vi "Time Profile Logger.vi"(6 "Flush and Close? (F)":bool, 7 "Initialize Settings":T1={"File Name"="SLL Time Profile Logger.txt", "Log Directory Path"=path "", "Initialize? (F)"=FALSE}, 8 "Error In":errorcluster, 9 "Tag Array":string[](array[string]), 10 "Tag 2":string, 11 "Tag 1":string) -> (0 "Error Out":errorcluster, 3 "Log Path":path)   [LabVIEW 2014, in "SLL Debug.lvlib"]
doc: "Simple Time Profile Logger with multiple tag inputs. \n\n<b>Important!</b> -The final call to this VI needs to have the \"Flush and Close?\" boolean set to log to file.\n\nDuring logging, the items are just put into a queue. Only during close operation, the data is parsed and logged to file. Supports logging into *.bin, *.csv & *.txt based on the file extension provided to the file name."
uses:
  SLL Debug.lvlib
  <vilib>/Utility/file.llb/Write To Spreadsheet File (string).vi
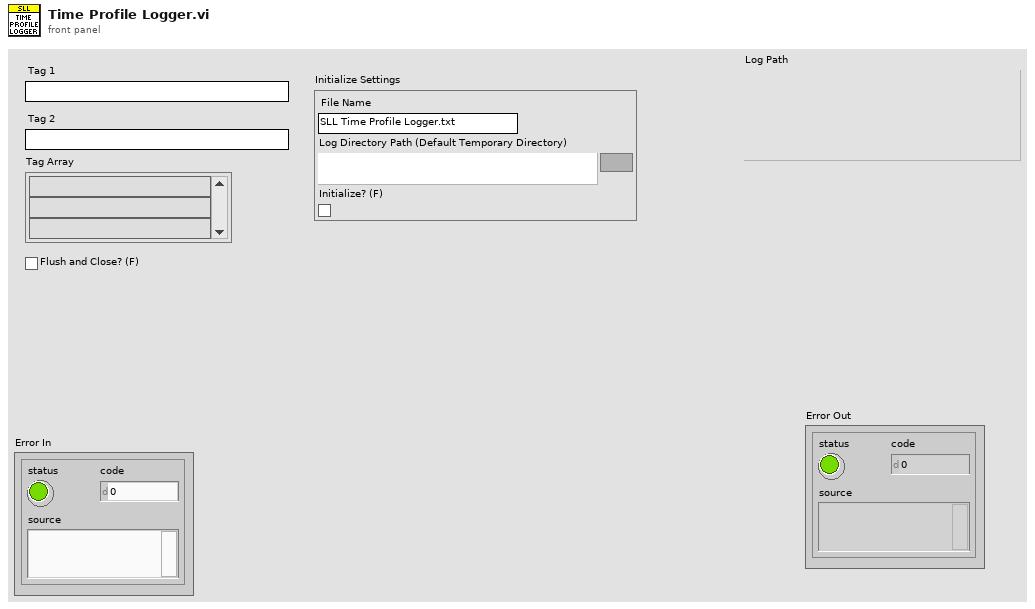
[diagram p1: front panel]
types:
  T1 = cluster{"File Name":string, "Log Directory Path":path, "Initialize? (F)":bool}
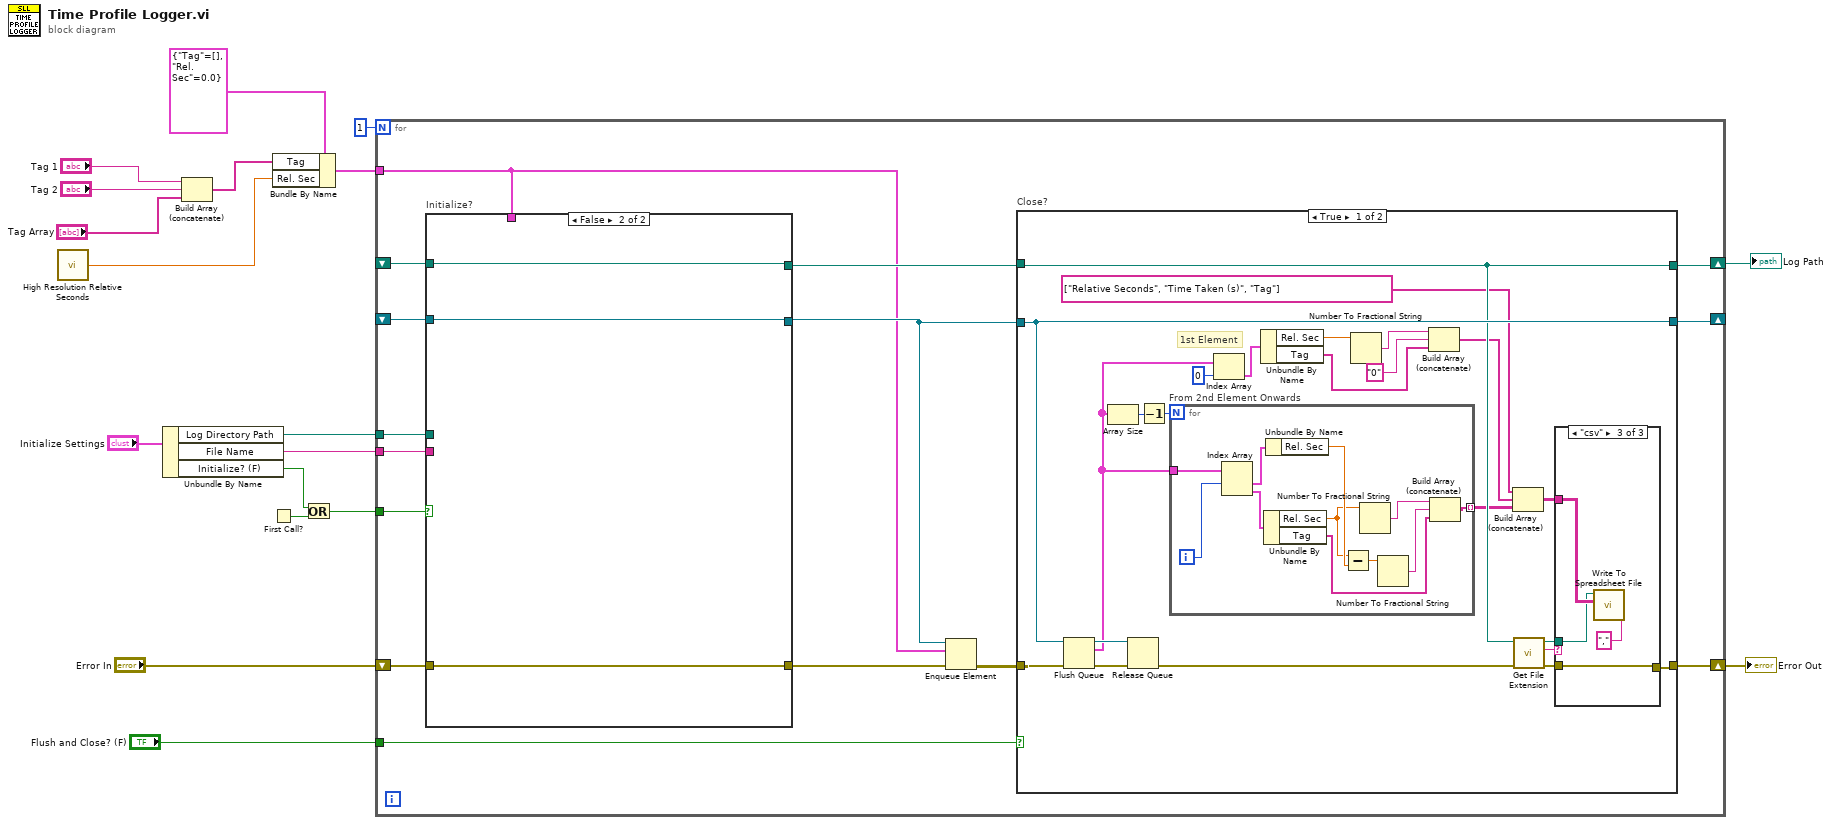
[diagram p0: block diagram]
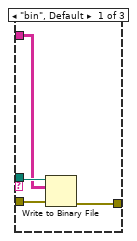
[diagram p2: hidden frame]
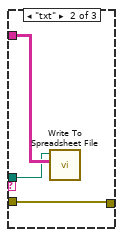
[diagram p3: hidden frame]
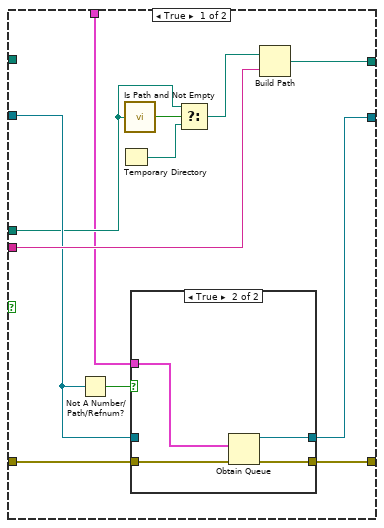
[diagram p5: hidden frame]
diagram:
  n1 = call <vilib>:"High Resolution Relative Seconds.vi"() -> ("relative seconds"=w2:dbl)
  n2 = Unbundle By Name("Initialize Settings") -> ("Log Directory Path"=w11:path, "File Name"=w10:string, "Initialize? (F)"=w6:bool)
  n3 = Build Array (concatenate)("Tag 1", "Tag 2", "Tag Array") -> (w4:string[])
  n4 = First Call?() -> (First Call?: T/F=w1:bool)
  n5 = Bundle By Name(cluster=cluster{"Tag":string[], "Rel. Sec":dbl} {"Tag"=[], "Rel. Sec"=0.0}, "Tag"=w4, "Rel. Sec"=w2) -> (w3:cluster{"Tag":string[], "Rel. Sec":dbl})
  n6 = Or(x=w6, y=w1) -> (x .or. y?=w9:bool)
  n7 = for {
    N: 1 -> [_]
    tunnel: w3 -> [w19]
    shift-right: [w20] -> w17
    shift-left: "Error In" -> [w33]
    shift-right: [w22] -> _
    shift-left: _ -> [w32]
    tunnel: w10 -> [w31]
    shift-right: [w21] -> w16
    shift-left: _ -> [w30]
    tunnel: w11 -> [w29]
    tunnel: w9 -> [w28]
    tunnel: "Flush and Close? (F)" -> [w27]
    n8 = case "Initialize?" shown="False" w28 {
      tunnel: w33 -> [w93 w102]
      tunnel: [w92 w102] -> w26
      tunnel: [w91 w101] -> w23
      tunnel: w32 -> [w87 w101]
      tunnel: w31 -> [w90 _]
      tunnel: [w89 w100] -> w24
      tunnel: w30 -> [_ w100]
      tunnel: w29 -> [w85 _]
      tunnel: w19 -> [w82 _]
      frame True {
        n9 = Not A Number/Path/Refnum?(number/path/refnum=w87) -> (NaN/Path/Refnum?=w88:bool)
        n10 = Temporary Directory() -> (w84:path)
        n11 = call <vilib>:"Is Path and Not Empty.vi"("path"=w85) -> ("Is Path and Not Empty?"=w86:bool)  [unwired: 4 in]
        n12 = case shown="True" w88 {
          tunnel: w93 -> [w94 w99]
          tunnel: [w94 w98] -> w92
          tunnel: [w95 w97] -> w91
          tunnel: w87 -> [w95 _]
          tunnel: w82 -> [_ w96]
          frame False {
          }
          frame True {
            n13 = Obtain Queue(element data type=w96, error in (no error)=w99) -> (queue out=w97:refnum<queue>, error out=w98:errorcluster)  [unwired: 3 in, 1 out]
          }
        }
        n14 = Select(t=w85, s=w86, f=w84) -> (s? t:f=w83:path)
        n15 = Build Path(base path=w83, name or relative path=w90) -> (appended path=w89:path)
      }
      frame False {
      }
    }
    n16 = Enqueue Element(queue=w23, element=w19, error in (no error)=w26) -> (error out=w25:errorcluster)  [unwired: 1 in, 2 out]
    n17 = case "Close?" shown="True" w27 {
      tunnel: w25 -> [w56 w81]
      tunnel: [w47 w81] -> w20
      tunnel: [w54 w80] -> w22
      tunnel: w23 -> [w54 w80]
      tunnel: [w51 w79] -> w21
      tunnel: w24 -> [w51 w79]
      frame True {
        # "1st Element"
        n18 = Flush Queue(queue=w54, error in (no error)=w56) -> (queue out=w53:refnum<queue>, remaining elements=w36:cluster{"Tag":string[], "Rel. Sec":dbl}[], error out=w55:errorcluster)
        n19 = Array Size(array=w36) -> (size(s)=w37:i32)
        n20 = Release Queue(queue=w53, error in (no error)=w55) -> (error out=w52:errorcluster)  [unwired: 1 in, 2 out]
        n21 = Decrement(x=w37) -> (x-1=w38:i32)
        n22 = for "From 2nd Element Onwards" {
          N: w38 -> [_]
          tunnel: w36 -> [w67]
          tunnel: [w61] -> w39 mode=indexing
          i -> [w66]
          n23 = Index Array(array=w67, index #1=w66) -> (element #1=w65:cluster{"Tag":string[], "Rel. Sec":dbl}, element #2=w64:cluster{"Tag":string[], "Rel. Sec":dbl})  [unwired: 1 in]
          n24 = Unbundle By Name(w64) -> ("Rel. Sec"=w59:dbl, "Tag"=w57:string[])
          n25 = Unbundle By Name(w65) -> ("Rel. Sec"=w63:dbl)
          n26 = Subtract(x=w59, y=w63) -> (x-y=w62:dbl)
          n27 = Number To Fractional String(number=w59) -> (F-format string=w58:string)  [unwired: 3 in]
          n28 = Number To Fractional String(number=w62) -> (F-format string=w60:string)  [unwired: 3 in]
          n29 = Build Array (concatenate)(w58, w60, w57) -> (w61:string[])
        }
        n30 = Index Array(array=w36, index=0) -> (element=w41:cluster{"Tag":string[], "Rel. Sec":dbl})
        n31 = Unbundle By Name(w41) -> ("Rel. Sec"=w42:dbl, "Tag"=w34:string[])
        n32 = Number To Fractional String(number=w42) -> (F-format string=w43:string)  [unwired: 3 in]
        n33 = Build Array (concatenate)(w43, "0", w34) -> (w46:string[])
        n34 = Build Array (concatenate)(string[] ["Relative Seconds", "Time Taken (s)", "Tag"], w46, w39) -> (w35:string[][])
        n35 = call <vilib>:"Get File Extension.vi"("error in (no error)"=w52, "file"=w51) -> ("error out"=w49:errorcluster, "lowercase file extension"=w50:string, "dup file"=w48:path)  [unwired: 6 in, 1 out]
        n36 = case shown="\"csv\"" w50 {
          tunnel: w35 -> [w68 w74 w78]
          tunnel: w49 -> [w70 w72 w76]
          tunnel: w48 -> [w71 w73 w77]
          tunnel: [w69 w72 w76] -> w47
          frame "bin", Default {
            n37 = Write to Binary File(file (use dialog)=w71, data=w68, error in=w70) -> (error out=w69:errorcluster)  [unwired: 3 in, 2 out]
          }
          frame "txt" {
            n38 = call-poly <vilib>:"Write To Spreadsheet File.vi"("2D data"=w74, "file path (dialog if empty)"=w73) -> ()  [unwired: 6 in, 1 out]
          }
          frame "csv" {
            n39 = call-poly <vilib>:"Write To Spreadsheet File.vi"("delimiter (\\t)"="," ("delimiter (\\t)"), "2D data"=w78, "file path (dialog if empty)"=w77) -> ()  [unwired: 5 in, 1 out]
          }
        }
      }
      frame False {
      }
    }
  }
  "Error Out" <- w17
  "Log Path" <- w16
